vi "Config-Chan-VSUs-Sampling.vi"(0 "VISA session":refnum<visa-resource-name>, 1 "VSU1 function":bool, 2 "VSU2 standby":bool, 5 "VSU1 standby":bool, 7 "VSU1 V name \n(max 6 chars)":string, 9 "VSU2 V name \n(max 6 chars)":string, 11 "error in (no error)":errorcluster, 12 "VSU2 function":bool) -> (4 "VISA resource name out":refnum<visa-resource-name>, 15 "error out":errorcluster)   [LabVIEW 2016, in "Agilent 415X Series.lvlib"]
doc: "This VI configures both VSUs in sweep measurement mode. \n\nThis VI corresponds to the Channel Definition Page (when Measurement Mode is set to SWEEP) of the instrument. In general, it allows every setting change that can be made via the instrument's front panel although the change may cause a setting conflict when a measurement is initialied."
uses:
  Agilent 415X Series.lvlib
panel:
  # "* This VI does NOT report all setting errors. Error \nchecking must be done when a measurement is initialized."
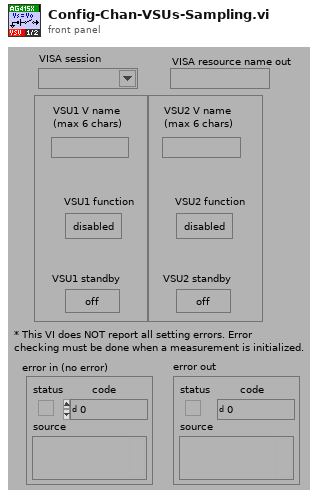
[diagram p1: front panel]
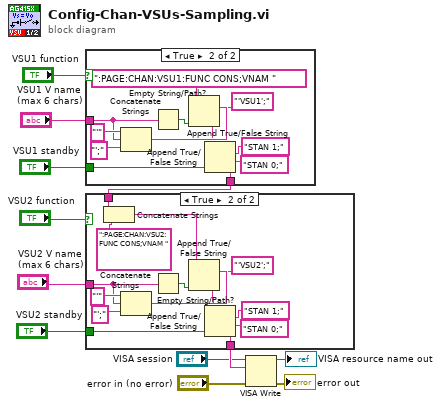
[diagram p0: block diagram]
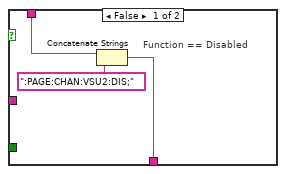
[diagram p2: hidden frame]
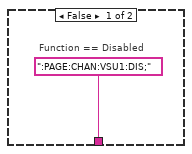
[diagram p3: hidden frame]
diagram:
  n1 = case shown="True" "VSU1 function" {
    tunnel: "VSU1 V name \n(max 6 chars)" -> [_ w23]
    tunnel: "VSU1 standby" -> [_ w18]
    tunnel: [":PAGE:CHAN:VSU1:DIS;" w19] -> w7
    frame False {
      # "Function == Disabled"
    }
    frame True {
      n2 = Concatenate Strings("'", w23, "';") -> (w22:string)
      n3 = Empty String/Path?(string/path=w23) -> (empty?=w25:bool)
      n4 = Append True/False String(1:w25, 2:w22, 3:"'VSU1';", 4:":PAGE:CHAN:VSU1:FUNC CONS;VNAM ") -> (0:w16:string)
      n5 = Append True/False String(1:w18, 2:"STAN 0;", 3:"STAN 1;", 4:w16) -> (0:w19:string)
    }
  }
  n6 = case shown="True" "VSU2 function" {
    tunnel: "VSU2 V name \n(max 6 chars)" -> [_ w40]
    tunnel: "VSU2 standby" -> [_ w35]
    tunnel: [w28 w36] -> w6
    tunnel: w7 -> [w26 w31]
    frame False {
      # "Function == Disabled"
      n7 = Concatenate Strings(w26, ":PAGE:CHAN:VSU2:DIS;") -> (w28:string)
    }
    frame True {
      n8 = Concatenate Strings(w31, ":PAGE:CHAN:VSU2:FUNC CONS;VNAM ") -> (w30:string)
      n9 = Concatenate Strings("'", w40, "';") -> (w39:string)
      n10 = Empty String/Path?(string/path=w40) -> (empty?=w42:bool)
      n11 = Append True/False String(1:w42, 2:w39, 3:"'VSU2';", 4:w30) -> (0:w33:string)
      n12 = Append True/False String(1:w35, 2:"STAN 0;", 3:"STAN 1;", 4:w33) -> (0:w36:string)
    }
  }
  n13 = VISA Write(VISA resource name="VISA session", write buffer=w6, error in (no error)="error in (no error)") -> (VISA resource name out=→"VISA resource name out":refnum<visa-resource-name>, error out=→"error out":errorcluster)  [unwired: 1 out]
